vi "ErrorHandle.vi"(8 "error in (no error)":errorcluster) -> (0 "error in (no error) 2":errorcluster)   [LabVIEW 2021]
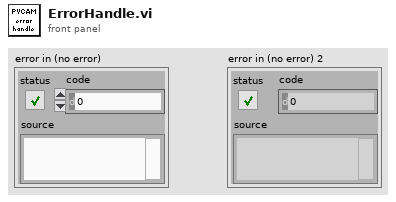
[diagram p1: front panel]
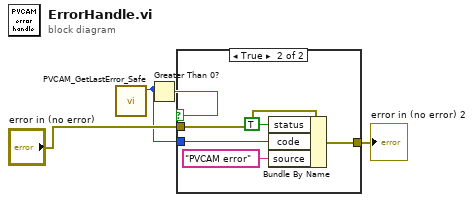
[diagram p0: block diagram]
diagram:
  n1 = call "PVCAM_GetLastError_Safe.vi"() -> ("return type"=w2:i16)  [unwired: 11 in]
  n2 = Greater Than 0?(x=w2) -> (x > 0?=w4:bool)
  n3 = case shown="True" w4 {
    tunnel: "error in (no error)" -> [w5 w10]
    tunnel: w2 -> [_ w8]
    tunnel: [w5 w6] -> w1
    frame False {
    }
    frame True {
      n4 = Bundle By Name(cluster=w10, "status"=TRUE, "code"=w8, "source"="PVCAM error") -> (w6:errorcluster)
    }
  }
  "error in (no error) 2" <- w1
